vi "Extract (no data).vi"(8 "error in (no error)":errorcluster, 11 "Message":refnum<class "MSG.lvclass">) -> (0 "error out":errorcluster, 2 "Label":string, 3 "Message":refnum<class "MSG.lvclass">)   [LabVIEW 2011, in "Messenging.lvlib" / "MSG.lvclass"]
uses:
  MSG.lvclass
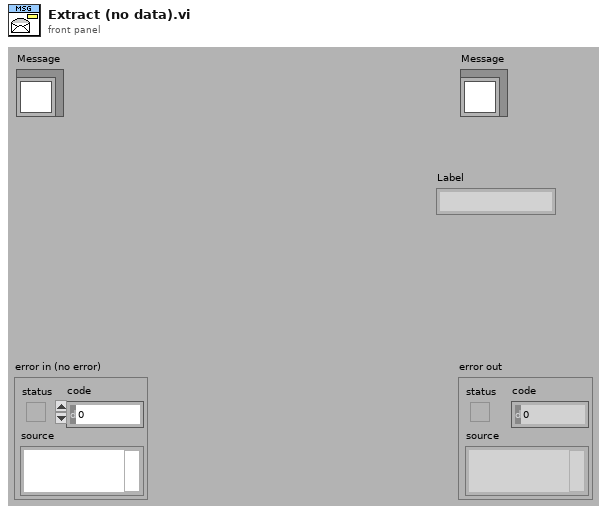
[diagram p1: front panel]
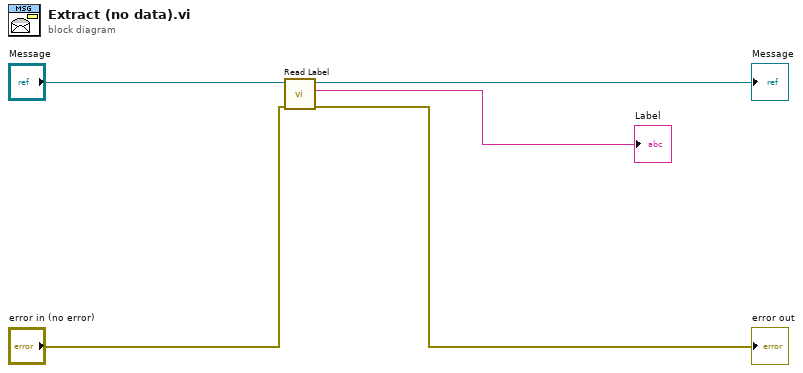
[diagram p0: block diagram]
diagram:
  n1 = call-dynamic "Read Label.vi"("error in (no error)"="error in (no error)", "Message"="Message") -> ("error out"=→"error out":errorcluster, "Label"=→"Label":string, "Message"=→"Message":refnum<class "MSG.lvclass">)  [unwired: 7 out]
